vi "rwfm_Stop.vi"(8 "error in":errorcluster, 11 "Dynamic FPGA VI Reference":T1) -> (0 "error out":errorcluster, 3 "Dynamic FPGA VI Reference":T1)   [LabVIEW 2017, in "cRIOWfmLib.lvlib"]
doc: "This VI sends a stop command to the FPGA's acquisition loop and waits for confirmation that the loop has indeed stopped. The VI also flushes the host's data buffer so subsequent acquisitions do not read old data."
uses:
  <vilib>/addons/InsightCM/Devices/Shared/Cms/cRIOWfmAcq/cRIOWfmLib.lvlib
  <vilib>/addons/InsightCM/Devices/Shared/Cms/cRIOWfmAcq/subVIs/RIO Wfm Cust Ctrls/rwfm_DynamicFPGAref2.ctl
  <vilib>/rvi/errors/niLvFpgaAdjustHostInterfaceError.vi
  <vilib>/rvi/interface/nirviReadWriteControl/nirviReadWriteControl.xnode
  <vilib>/rvi/interface/nirviMethod/nirviMethod.xnode
  NiFpgaLv.dll
  <vilib>/rvi/interface/Simulation/niFpgaSimulationCallBeginRW.vi
  <vilib>/FPGAPlugInAG/Dynamic/niLvFpga_ReadFifo_Dynamic.vi
  <vilib>/rvi/errors/niLvFpgaMergeErrorWithErrorCode.vi
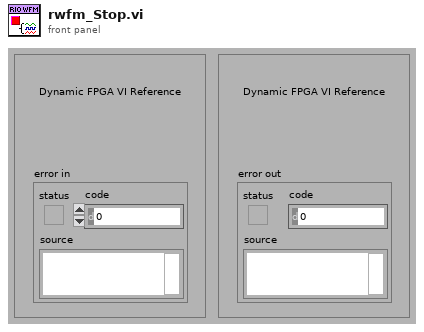
[diagram p1: front panel]
types:
  T1 = typedef "cRIOWfmLib.lvlib/rwfm_DynamicFPGAref2.ctl" = refnum<k20>
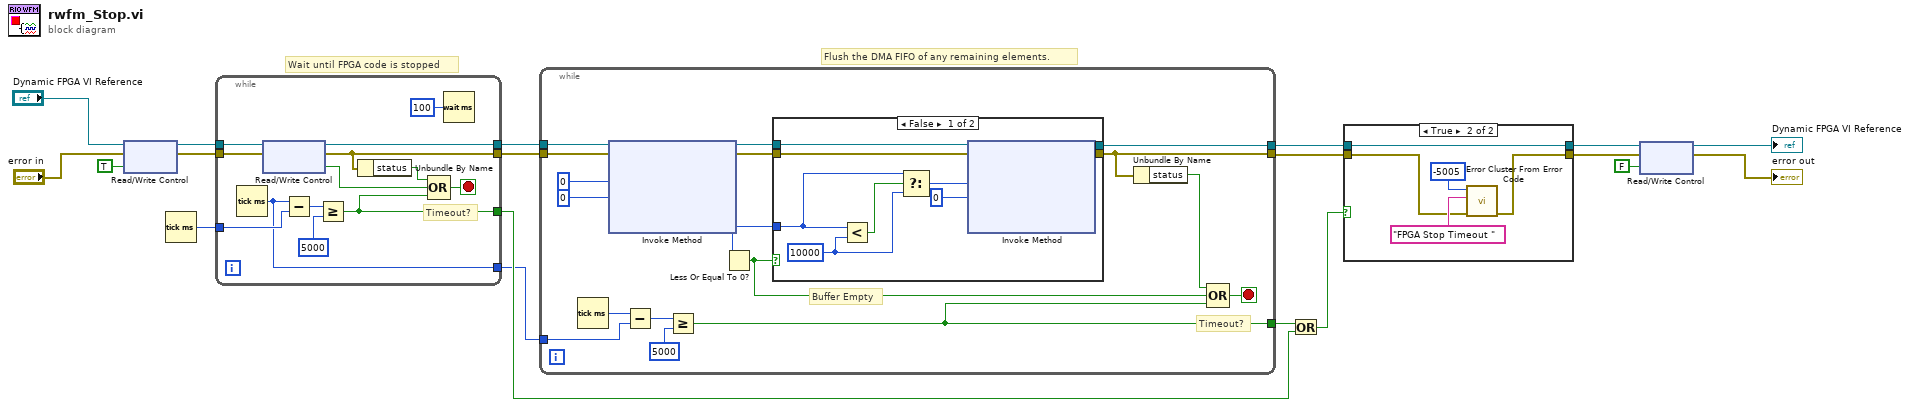
[diagram p0: block diagram]
diagram:
  # "Wait until FPGA code is stopped"
  # "Flush the DMA FIFO of any remaining elements."
  n1 = xnode "Read/Write Control"("FPGA VI Reference In"="Dynamic FPGA VI Reference", "error in"="error in", "Stop"=TRUE) -> ("FPGA VI Reference Out"=w17:T1, "error out"=w16:errorcluster)
  n2 = Tick Count (ms)() -> (millisecond timer value=w9:u32)
  n3 = while {
    tunnel: w17 -> [w32]
    tunnel: w16 -> [w31]
    tunnel: [w29] -> w15
    tunnel: [w25] -> w14
    tunnel: w9 -> [w28]
    tunnel: [w22] -> w7
    tunnel: [w21] -> w5
    stop <- w23 stop-if-true
    # "Timeout?"
    n4 = Tick Count (ms)() -> (millisecond timer value=w21:u32)
    n5 = xnode "Read/Write Control"("FPGA VI Reference In"=w32, "error in"=w31) -> ("FPGA VI Reference Out"=w29:T1, "error out"=w25:errorcluster, "Finished"=w20:bool)
    n6 = Subtract(x=w21, y=w28) -> (x-y=w27:u32)
    n7 = Greater Or Equal?(x=w27, y=u32 5000) -> (x >= y?=w22:bool)
    n8 = Unbundle By Name(w25) -> ("status"=w24:bool)
    n9 = Compound Arithmetic op=OR(w24, w20, w22) -> (w23:bool)
    n10 = Wait (ms)(milliseconds to wait=u32 100) -> ()  [unwired: 1 out]
  }
  n11 = while {
    tunnel: [w47] -> w13
    tunnel: [w44] -> w10
    tunnel: w15 -> [w46]
    tunnel: w14 -> [w45]
    tunnel: w5 -> [w37]
    tunnel: [w36] -> w8
    stop <- w42 stop-if-true
    # "Timeout?"
    # "Buffer Empty"
    n12 = Tick Count (ms)() -> (millisecond timer value=w38:u32)
    n13 = xnode "Invoke Method"("FPGA VI Reference In"=w46, "error in"=w45, "Number of Elements"=u32 0, "Timeout (ms)"=0) -> ("FPGA VI Reference Out"=w49:T1, "error out"=w48:errorcluster, "Elements Remaining"=w33:u32)  [unwired: 1 out]
    n14 = Subtract(x=w38, y=w37) -> (x-y=w39:u32)
    n15 = Greater Or Equal?(x=w39, y=u32 5000) -> (x >= y?=w36:bool)
    n16 = Less Or Equal To 0?(x=w33) -> (x <= 0?=w41:bool)
    n17 = case shown="False" w41 {
      tunnel: w49 -> [w58 w60]
      tunnel: w48 -> [w57 w59]
      tunnel: [w56 w60] -> w47
      tunnel: [w55 w59] -> w44
      tunnel: w33 -> [w52 _]
      frame False {
        w53 = u32 10000
        n18 = Less?(x=w52, y=w53) -> (x < y?=w54:bool)
        n19 = Select(t=w52, s=w54, f=w53) -> (s? t:f=w51:u32)
        n20 = xnode "Invoke Method"("FPGA VI Reference In"=w58, "error in"=w57, "Number of Elements"=w51, "Timeout (ms)"=0) -> ("FPGA VI Reference Out"=w56:T1, "error out"=w55:errorcluster)  [unwired: 2 out]
      }
      frame True {
      }
    }
    n21 = Unbundle By Name(w44) -> ("status"=w43:bool)
    n22 = Compound Arithmetic op=OR(w43, w41, w36) -> (w42:bool)
  }
  n23 = Or(x=w8, y=w7) -> (x .or. y?=w6:bool)
  n24 = case shown="True" w6 {
    tunnel: [w62 w67] -> w12
    tunnel: w13 -> [w62 w67]
    tunnel: w10 -> [w61 w64]
    tunnel: [w61 w63] -> w11
    frame False {
    }
    frame True {
      n25 = call <vilib>:"Error Cluster From Error Code.vi"("error in (no error)"=w64, "error message (\"\")"="FPGA Stop Timeout " ("error message (\"\")"), "error code (0)"=-5005) -> ("error out"=w63:errorcluster)  [unwired: 1 in, 5 out]
    }
  }
  n26 = xnode "Read/Write Control"("FPGA VI Reference In"=w12, "error in"=w11, "Stop"=FALSE) -> ("FPGA VI Reference Out"=→"Dynamic FPGA VI Reference":T1, "error out"=→"error out":errorcluster)
